vi "Close Osciloscope.vi"(8 "error in (no error)":errorcluster, 11 "EDU-X 1002A in":refnum<class "EDU-X 1002A.lvclass">) -> (0 "error out":errorcluster, 3 "EDU-X 1002A out":refnum<class "EDU-X 1002A.lvclass">)   [LabVIEW 2020, in "EDU-X 1002A.lvclass"]
uses:
  EDU-X 1002A.lvclass
  C:/Users/HP/Desktop/Osciloscope/Class/OsciloscopeClass/OsciloscopeClass.lvclass
  OsciloscopeClass/OsciloscopeClass.lvclass/OsciloscopeClass.ctl
  OsciloscopeClass/Read Com Port.vi
  EDU-X 1002A.lvclass/EDU-X 1002A.ctl
  <instrlib>/Agilent 2000 3000 X-Series/Agilent 2000 3000 X-Series.lvlib
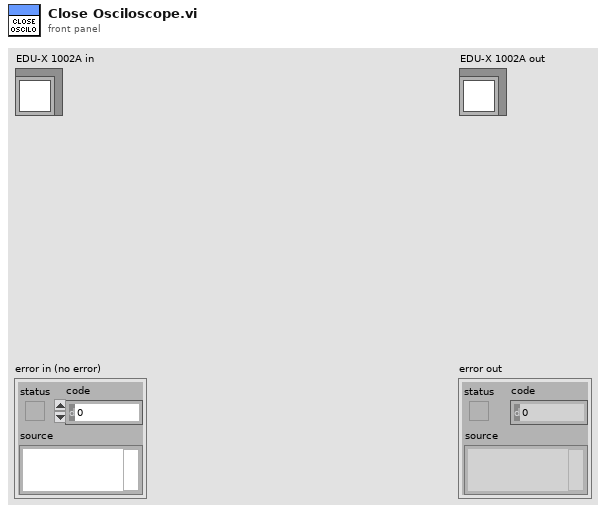
[diagram p1: front panel]
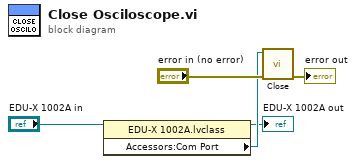
[diagram p0: block diagram]
diagram:
  n1 = property class="EDU-X 1002A.lvclass"(reference="EDU-X 1002A in") -> (reference out=→"EDU-X 1002A out":refnum<class "EDU-X 1002A.lvclass">, "Accessors:Com Port"=w2:refnum<visa-resource-name>)  [unwired: 1 in, 1 out]
  n2 = call <instrlib>:"Close.vi"("error in (no error)"="error in (no error)", "VISA resource name"=w2) -> ("error out"=→"error out":errorcluster)  [unwired: 9 in]
